vi "TestMotorCommands.vi"() -> ()   [LabVIEW 2017]
uses:
  LV_Source/Subsystems/Motion/DataTypes/Motion Settings--cluster.ctl
  Ichor_Common/Lib/Serial/Comm Channels--cluster.ctl
  Ichor_Common/Lib/Serial/SerialPort Config--cluster.ctl
  Ichor_Common/Lib/SmartMotor/TD SerialBusMotorSpecifier_enum.ctl
  Ichor_Common/Lib/SmartMotor/TD MotorCommands - single motor--enum.ctl
  LV_Source/Subsystems/Motion/Motion.lvclass
panel:
  out "str out 4":string[](array[string])
  out "cmdstr out 4":string[](array[string])
  in  "Rsp?":bool
  out "AdHoc Rsp":string
  in  "AdHoc Cmd":string
  in  "SendAdHoc":bool
  in  "ID":bool
  out "Motor ID":string
  out "str out 3":string[](array[string])
  out "cmdstr out 3":string[](array[string])
  out "str out 2":string[](array[string])
  out "cmdstr out 2":string[](array[string])
  in  "Move":bool
  in  "OK":bool
  in  "MotorSpecifier(None)":T1=enum."M2"
  out "error out":errorcluster
  in  "error in (no error)":errorcluster
  in  "Motion Settings":T2={"Simulate"=FALSE, "SerialPort"=enum."COM3", "SerPort Config"={"termChar"=10, "timeout"=10000, "baud"=9600, "data bits"=8, "parity"=enum."None", "stop bits"=10, "flow control (0:none)"=0}, "MotorStartupCmds"=["€SADDR1", "ECHO", "SLEEP", "€SADDR2", "‚ECHO", "€WAKE"], "EnableTermChar"=FALSE, "MotorSyncTimeout_s"=0.0} {"SerPort Config"."flow control (0:none)" items=["None", "XON/XOFF", "RTS/CTS", "XON/XOFF & RTS/CTS", "DTR/DSR", "XON/XOFF & DTR/DSR"]; "SerPort Config"."stop bits" items=["1.0"=10, "1.5"=15, "2.0"=20]; "SerPort Config"."data bits" min=5 max=8 step=1; "SerPort Config"."termChar" format="%.0x"}
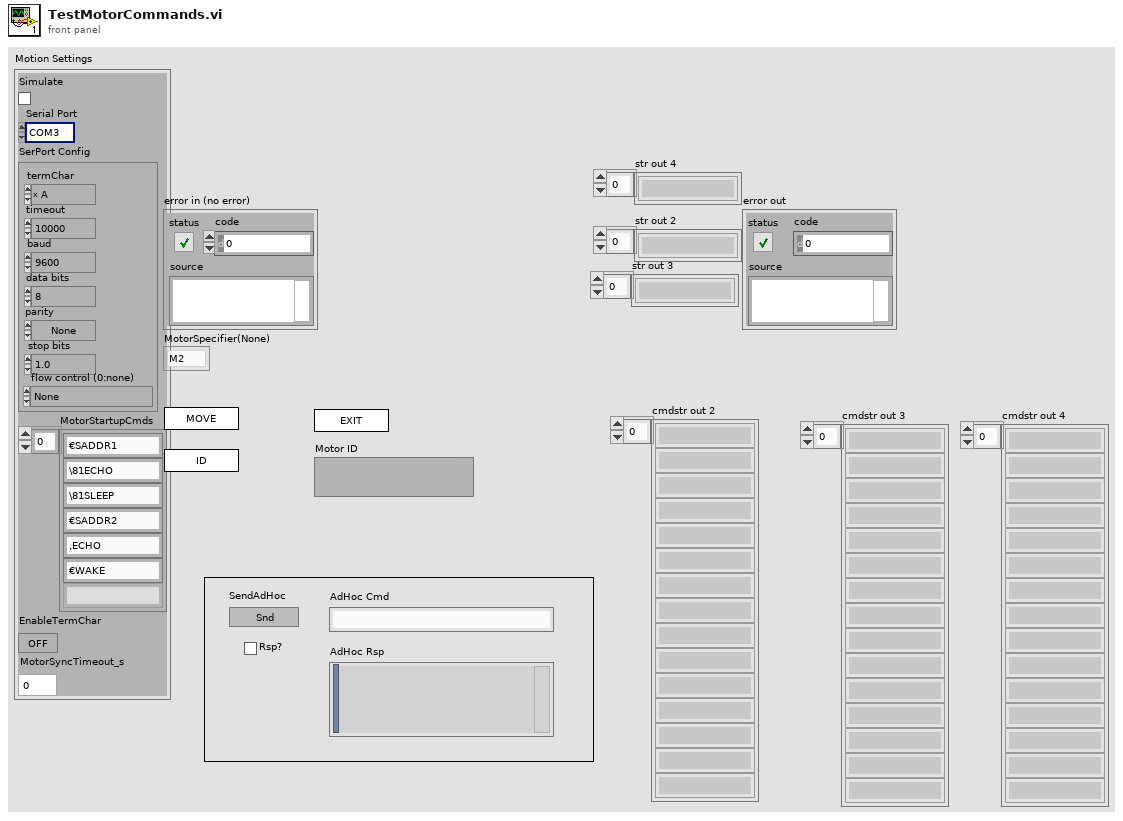
[diagram p1: front panel]
types:
  T1 = typedef "TD SerialBusMotorSpecifier_enum.ctl" = enum16{"None", "Global", "M1", "M2", "M3"}
  T2 = typedef "Motion.lvclass/Motion Settings--cluster.ctl" = cluster{"Simulate":bool, "SerialPort":T3, "SerPort Config":T4, "MotorStartupCmds":string[], "EnableTermChar":bool, "MotorSyncTimeout_s":dbl}
  T3 = typedef "Comm Channels--cluster.ctl" = enum16{"COM1", "COM2", "COM3", "COM4", "COM5", "COM6", "COM7", "COM8", "COM9", "COM10", "COM11", "COM12", "nothing", "LPT1", "LPT2", "LPT3", "LPT4"}
  T4 = typedef "SerialPort Config--cluster.ctl" = cluster{"termChar":u8, "timeout":u32, "baud":u32, "data bits":u16, "parity":enum16{"None", "Odd", "Even", "Mark", "Space"}, "stop bits":u16, "flow control (0:none)":u16}
  T5 = enum32{"invalid app kind", "Development System", "Run Time System", "Student Edition", "Embedded LabVIEW", "Evaluation", "Custom"}
  T6 = enum32{"Invalid", "Standard", "Closed", "Hidden", "Minimized", "Maximized"}
  T7 = typedef "TD MotorCommands - single motor--enum.ctl" = enum16{"Unlisted", "AbortMotion", "StopMotion", "DisableMotor", "ClearErrors", "ZeroEncoder", "SetMode", "GO", "SetEncoder", "En/Ds LmtSwitchs"}
  T8 = cluster{"String Input":string, "ExpectResponse":bool}
  T9 = cluster{"Core":cluster{"Current VI Reference":refnum<vi>, "Close Panel on Exit?":bool}, "VISA":refnum<visa-resource-name>}
  T10 = cluster{"Current VI Reference":refnum<vi>, "Close Panel on Exit?":bool}
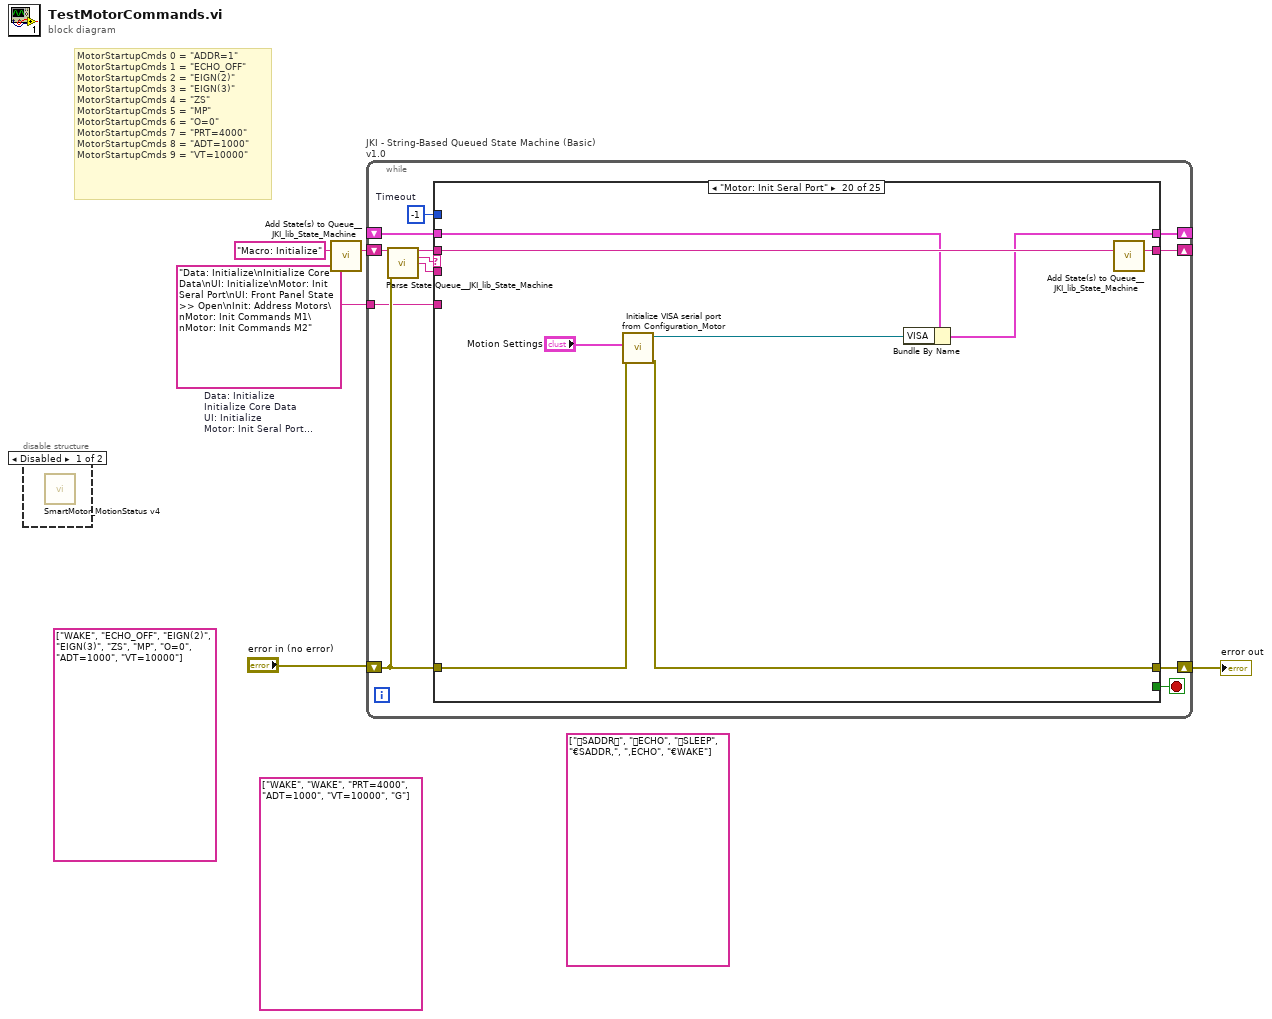
[diagram p0: block diagram]
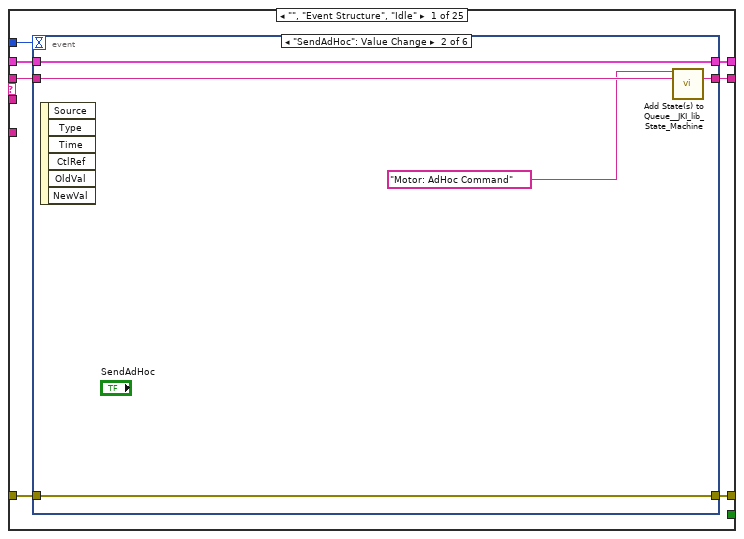
[diagram p3: hidden frame]
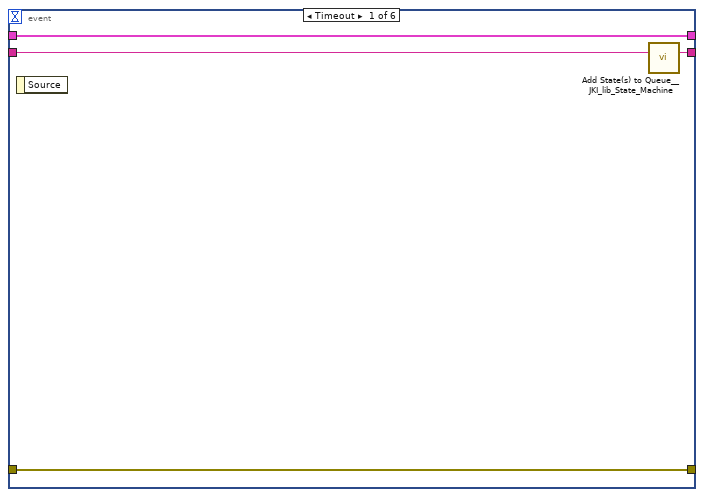
[diagram p4: hidden frame]
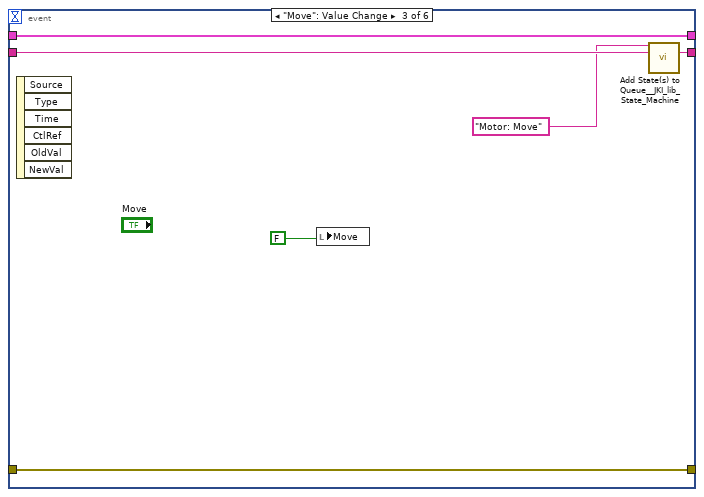
[diagram p5: hidden frame]
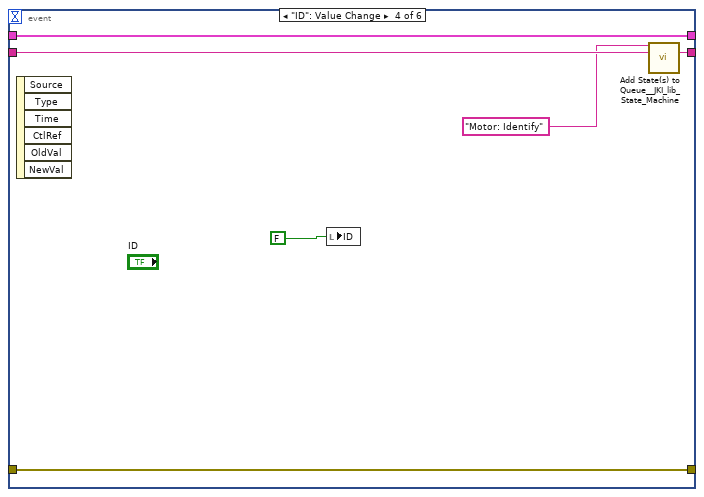
[diagram p6: hidden frame]
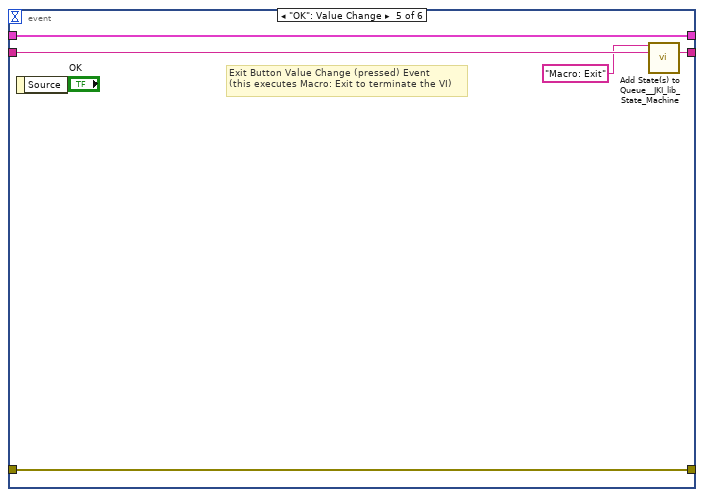
[diagram p7: hidden frame]
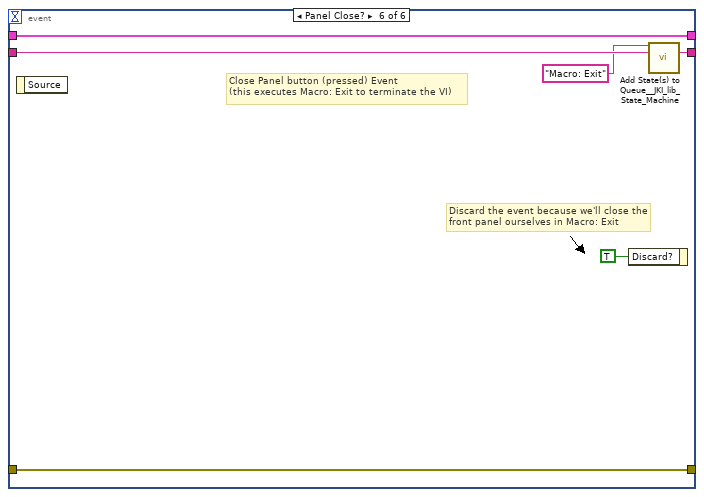
[diagram p8: hidden frame]
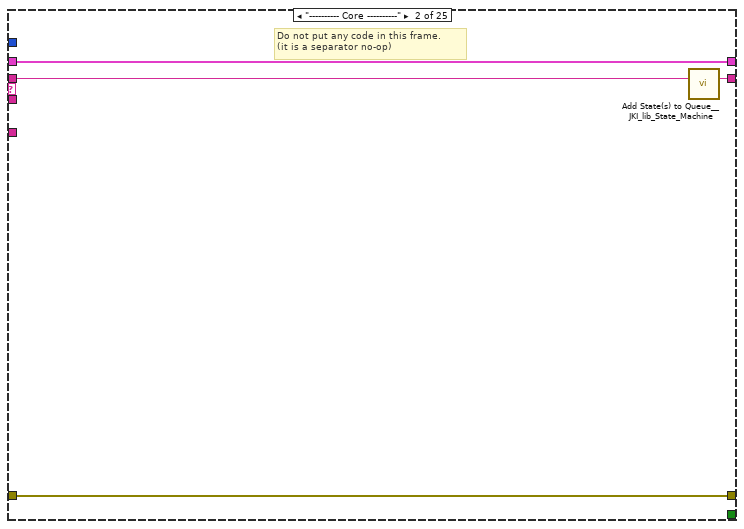
[diagram p9: hidden frame]
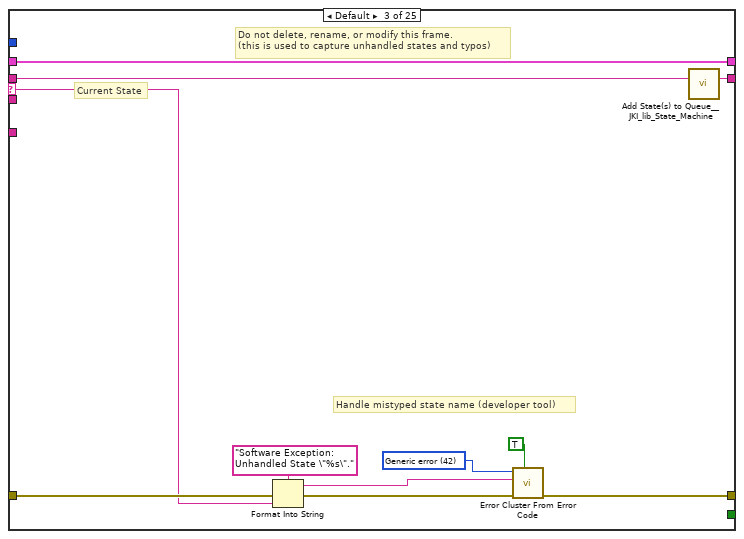
[diagram p10: hidden frame]
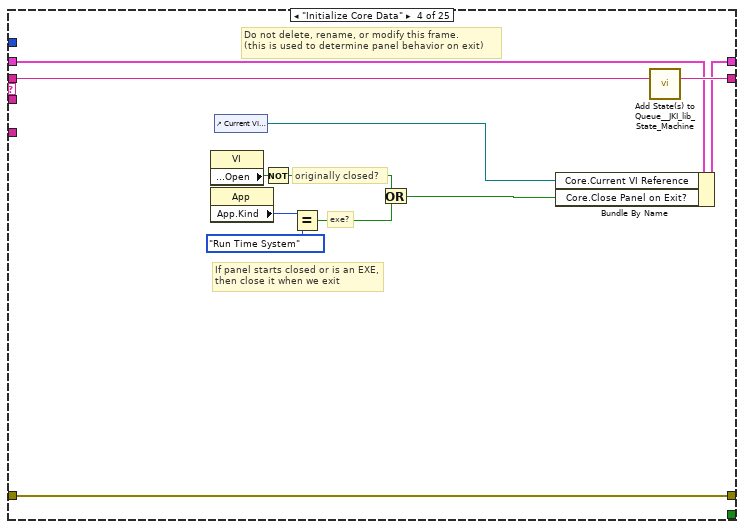
[diagram p11: hidden frame]
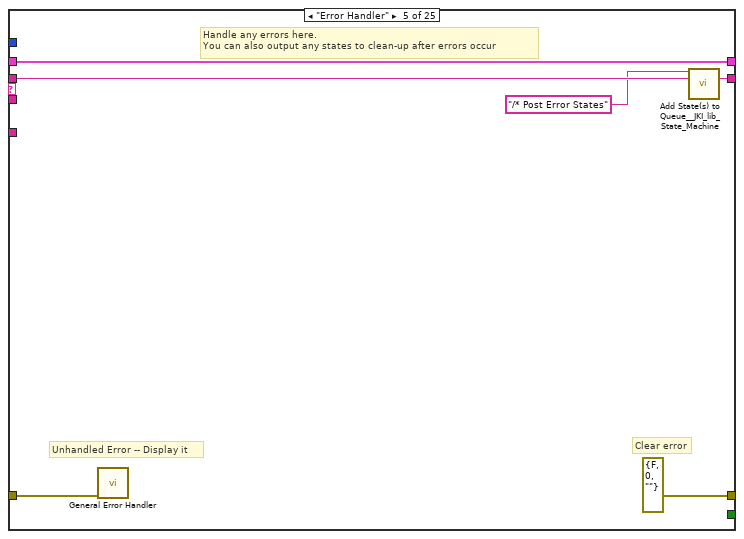
[diagram p12: hidden frame]
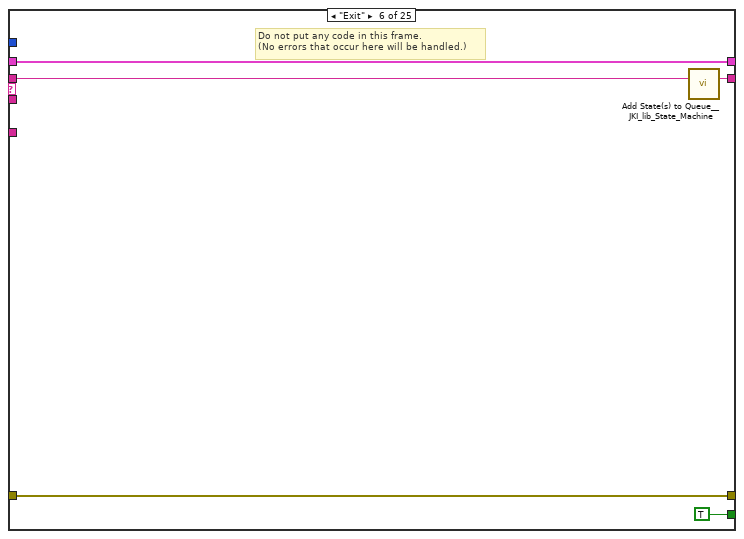
[diagram p13: hidden frame]
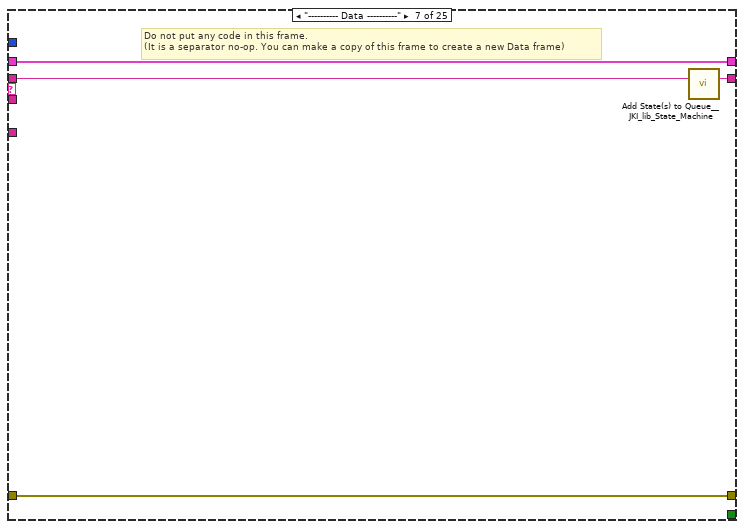
[diagram p14: hidden frame]
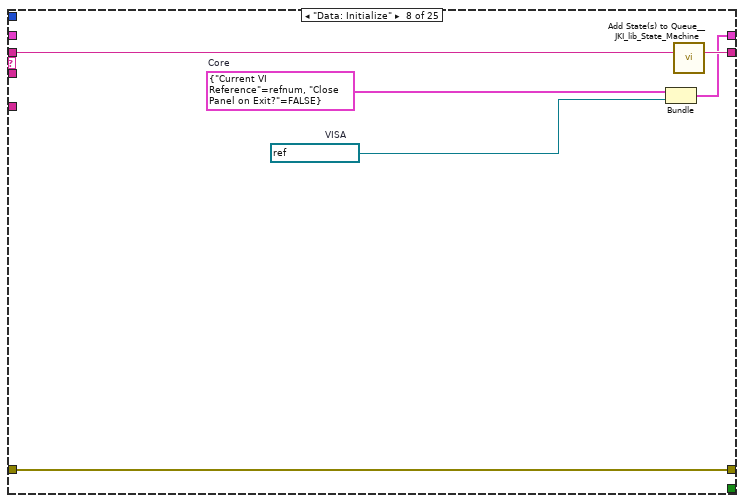
[diagram p15: hidden frame]
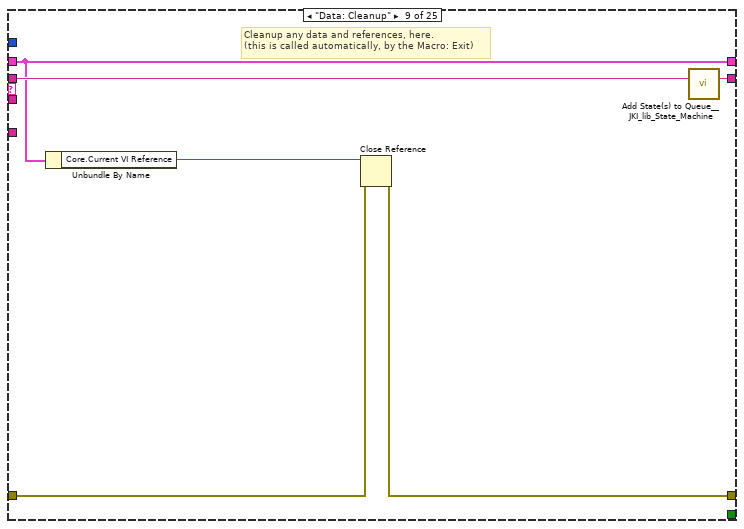
[diagram p16: hidden frame]
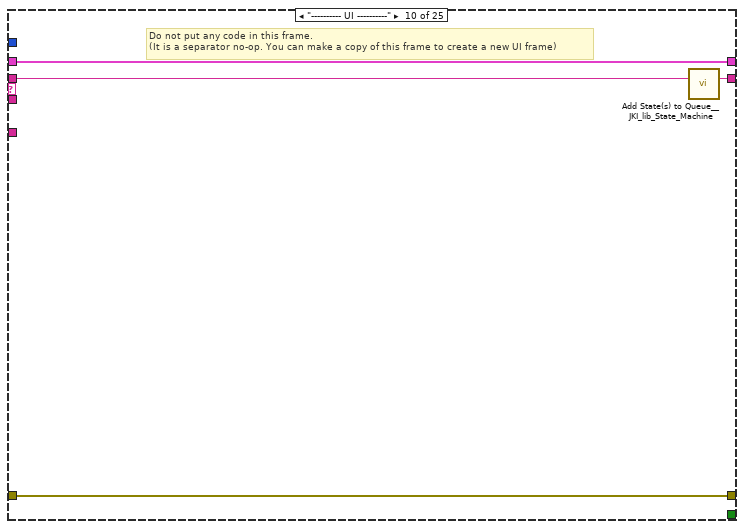
[diagram p17: hidden frame]
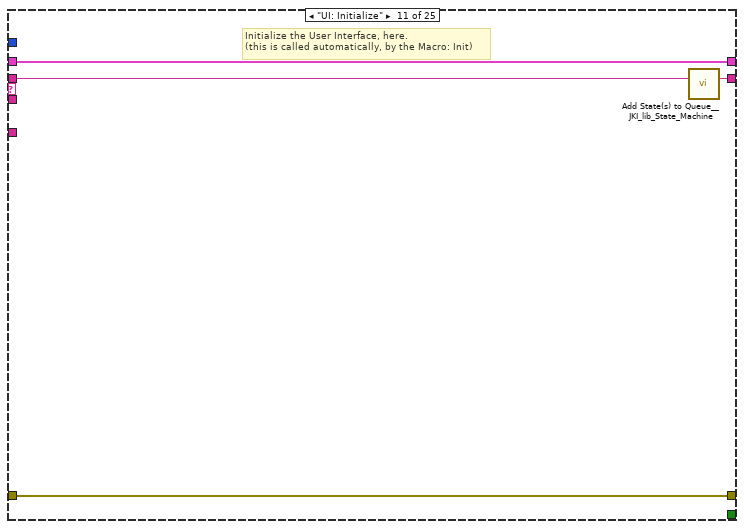
[diagram p18: hidden frame]
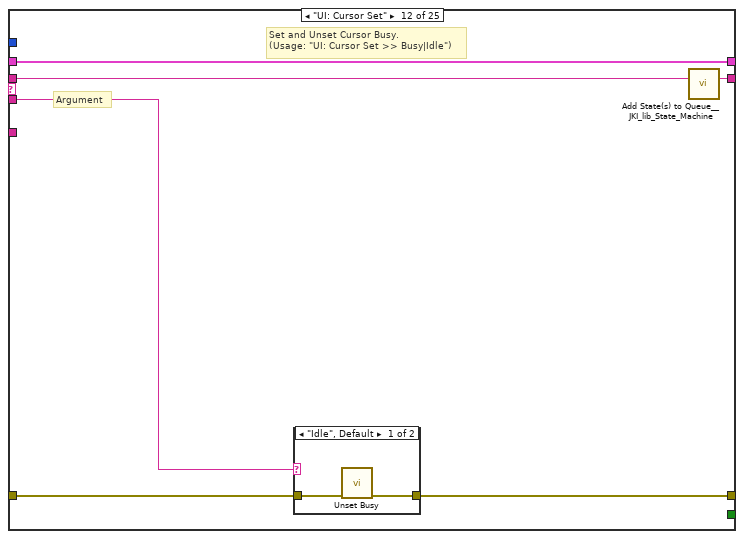
[diagram p19: hidden frame]
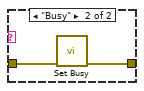
[diagram p20: hidden frame]
diagram:
  (unwired) string[] ["SADDR", "ECHO", "SLEEP", "€SADDR‚", "‚ECHO", "€WAKE"]
  (unwired) string[] ["WAKE", "WAKE", "PRT=4000", "ADT=1000", "VT=10000", "G"]
  (unwired) string[] ["WAKE", "ECHO_OFF", "EIGN(2)", "EIGN(3)", "ZS", "MP", "O=0", "ADT=1000", "VT=10000"]
  w1 = "Data: Initialize\nInitialize Core Data\nUI: Initialize\nMotor: Init Seral Port\nUI: Front Panel State >> Open\nInit: Address Motors\nMotor: Init Commands M1\nMotor: Init Commands M2"  # Data: Initialize Initialize Core Data UI: Initialize Motor: Init Seral Port UI: Front Panel State >> Open Init: Address Motors Motor: Init Commands M1 Motor: Init Commands M2
  # "MotorStartupCmds 0 = \"ADDR=1\"\nMotorStartupCmds 1 = \"ECHO_OFF\"\nMotorStartupCmds 2 = \"EIGN(2)\"\nMotorStartupCmds 3 = \"EIGN(3)\"\nMotorStartupCmds 4 = \"ZS\"\nMotorStartupCmds 5 = \"MP\"\nMotorStartupCmds 6 = \"O=0\"\nMotorStartupCmds 7 = \"PRT=4000\"\nMotorStartupCmds 8 = \"ADT=1000\"\nMotorStartupCmds 9 = \"VT=10000\""
  n1 = disable-structure shown="Disabled" {
    frame Disabled {
      n2 = call "SmartMotor_MotionStatus v4.vi"() -> ()  [unwired: 10 in, 6 out]
    }
    frame Enabled {
    }
  }
  n3 = call <vilib>:"Add State(s) to Queue__JKI_lib_State_Machine.vi"("State(s) in (\"\")"="Macro: Initialize") -> ("States Out"=w5:string)  [unwired: 14 in]
  n4 = while "JKI - String-Based Queued State Machine (Basic) v1.0" {
    shift-right: [w10] -> _
    shift-left: _ -> [w9]
    shift-right: [w13] -> w2
    shift-left: "error in (no error)" -> [w7]
    shift-right: [w12] -> _
    shift-left: w5 -> [w14]
    tunnel: w1 -> [w6]
    stop <- w11 stop-if-true
    w8 = -1  # Timeout
    n5 = call <vilib>:"Parse State Queue__JKI_lib_State_Machine.vi"("State Queue"=w14, "Error In (no error)"=w7) -> ("Remaining States"=w16:string, "Current State"=w17:string, "Arguments"=w15:string)  [unwired: 11 in]
    n6 = case shown="\"Motor: Init Seral Port\"" w17 {
      selector: w17 -> [_ _ w61 _ _ _ _ _ _ _ _ _ _ _ _ _ _ _ _ _ _ _ _ _ _]
      tunnel: w16 -> [w24 w60 w65 w83 w89 w94 w98 w104 w110 w114 w118 w124 w135 w161 w166 w176 w180 w194 w200 w208 w220 w246 w255 w276 w297]
      tunnel: w15 -> [_ _ _ _ _ _ _ _ _ _ _ w119 w129 _ _ _ _ _ _ _ _ _ _ _ _]
      tunnel: w9 -> [w22 w57 w63 w74 w86 w92 w95 _ w105 w111 w116 w122 w131 w158 w163 w173 w177 w192 w196 w205 w213 w241 w250 w271 w292]
      tunnel: [w21 w58 w67 w80 errorcluster {"status"=FALSE, "code"=0, "source"=""} ("error out") w91 w96 w101 w106 w112 w115 w120 w132 w159 w164 w174 w178 w187 w197 w201 w215 w243 w248 w269 w290] -> w13
      tunnel: w7 -> [w20 w58 w66 w80 w85 w91 w96 w101 w107 w112 w115 w121 w133 w159 w164 w174 w178 w188 w198 w202 w214 w242 w247 w268 w289]
      tunnel: [w23 w59 w64 w82 w88 w93 w97 w103 w109 w113 w117 w123 w134 w160 w165 w175 w179 w193 w199 w207 w219 w245 w254 w275 w296] -> w12
      tunnel: [_ _ _ _ _ TRUE _ _ _ _ _ _ _ _ _ _ _ _ _ _ _ _ _ _ _] -> w11
      tunnel: [w19 w57 w63 w81 w86 w92 w95 w102 w105 w111 w116 w122 w131 w158 w163 w173 w177 w192 w196 w204 w212 w240 w250 w271 w292] -> w10
      tunnel: w8 -> [w18 _ _ _ _ _ _ _ _ _ _ _ _ _ _ _ _ _ _ _ _ _ _ _ _]
      tunnel: w6 -> [_ _ _ _ _ _ _ _ _ _ _ _ _ _ w162 _ _ _ _ _ _ _ _ _ _]
      frame "", "Event Structure", "Idle" {
        n7 = event shown="[1] \"SendAdHoc\": Value Change" {
          selector: _ -> [_ _ _ _ _ _]
          dyn-events: _ -> [_ _ _ _ _ _]
          timeout: w18 -> [_ _ _ _ _ _]
          tunnel: w24 -> [w28 w33 w39 w45 w50 w56]
          tunnel: [w27 w32 w38 w44 w49 w55] -> w23
          tunnel: w22 -> [w25 w30 w36 w42 w47 w53]
          tunnel: [w26 w31 w37 w43 w48 w54] -> w21
          tunnel: w20 -> [w26 w31 w37 w43 w48 w54]
          tunnel: [w25 w30 w36 w42 w47 w53] -> w19
          event Timeout {
            n8 = event-data() -> ()  [unwired: 1 in, 1 out]
            n9 = call <vilib>:"Add State(s) to Queue__JKI_lib_State_Machine.vi"("State(s) in (\"\")"=w28) -> ("States Out"=w27:string)  [unwired: 14 in]
          }
          event "SendAdHoc": Value Change {
            n10 = event-data() -> ()  [unwired: 1 in, 6 out]
            n11 = call <vilib>:"Add State(s) to Queue__JKI_lib_State_Machine.vi"("State(s) in Front (\"\")"="Motor: AdHoc Command", "State(s) in (\"\")"=w33) -> ("States Out"=w32:string)  [unwired: 13 in]
          }
          event "Move": Value Change {
            n12 = event-data() -> ()  [unwired: 1 in, 6 out]
            n13 = local write "Move"(FALSE ("Move")) -> ()
            n14 = call <vilib>:"Add State(s) to Queue__JKI_lib_State_Machine.vi"("State(s) in Front (\"\")"="Motor: Move" ("State(s) in Front (\"\")"), "State(s) in (\"\")"=w39) -> ("States Out"=w38:string)  [unwired: 13 in]
          }
          event "ID": Value Change {
            n15 = event-data() -> ()  [unwired: 1 in, 6 out]
            n16 = local write "ID"(FALSE ("Move")) -> ()
            n17 = call <vilib>:"Add State(s) to Queue__JKI_lib_State_Machine.vi"("State(s) in Front (\"\")"="Motor: Identify" ("State(s) in Front (\"\")"), "State(s) in (\"\")"=w45) -> ("States Out"=w44:string)  [unwired: 13 in]
          }
          event "OK": Value Change {
            # "Exit Button Value Change (pressed) Event\n(this executes Macro: Exit to terminate the VI)"
            n18 = event-data() -> ()  [unwired: 1 in, 1 out]
            n19 = call <vilib>:"Add State(s) to Queue__JKI_lib_State_Machine.vi"("State(s) in Front (\"\")"="Macro: Exit", "State(s) in (\"\")"=w50) -> ("States Out"=w49:string)  [unwired: 13 in]
          }
          event Panel Close? {
            # "Discard the event because we'll close the front panel ourselves in Macro: Exit"
            # "Close Panel button (pressed) Event\n(this executes Macro: Exit to terminate the VI)"
            n20 = event-data() -> ()  [unwired: 1 in, 1 out]
            n21 = event-data("Discard?"=TRUE) -> ()  [unwired: 1 in, 1 out]
            n22 = call <vilib>:"Add State(s) to Queue__JKI_lib_State_Machine.vi"("State(s) in Front (\"\")"="Macro: Exit", "State(s) in (\"\")"=w56) -> ("States Out"=w55:string)  [unwired: 13 in]
          }
        }
      }
      frame "---------- Core ----------" {
        # "Do not put any code in this frame.\n(it is a separator no-op)"
        n23 = call <vilib>:"Add State(s) to Queue__JKI_lib_State_Machine.vi"("State(s) in (\"\")"=w60) -> ("States Out"=w59:string)  [unwired: 14 in]
      }
      frame Default {
        w70 = 42 items=["No error", "Argument error", "Memory is full", "Out of zone", "End of file", "File already open", "Generic file I/O error", "File not found", "File permission error", "Disk is full", "Duplicate path", "Too many files open", "System feature not enabled", "Resource file not found", "Cannot add resource", "Resource not found", "Image not found", "Image memory error", "Pen does not exist", "Config type invalid", "Config token not found", "Config parse error", "Config memory error", "Bad external code format", "Bad external code offset", "External code not present", "Null window", "Destroy window error", "Null menu", "Print aborted", "Bad print record", "Print driver error", "Windows error during printing", "Memory error during printing", "Print dialog error", "Generic print error", "Invalid device refnum", "Device not found", "Device parameter error", "Device unit error", "Cannot open device", "Device call aborted", "Generic error", "Cancelled by user", "Object ID too low", "Object ID too high", "Object not in heap", "Unknown heap", "Unknown object (invalid DefProc)", "Unknown object (DefProc not in table)", "Message out of range", "Invalid (null) method", "Unknown message", "Manager call not supported", "Bad address", "Network operation in progress", "Network operation timed out", "Connection is busy", "Network attribute not supported", "Network error", "Address in use", "System out of memory", "Connection aborted", "Connection refused", "Not connected", "Already connected", "Connection closed", "Initialization error (interapplication manager)", "Bad occurrence", "Wait on unbound occurrence handler", "Occurrence queue overflow", "Datalog type conflict", "Unused", "Unrecognized type (interapplication manager)", "Memory corrupt", "Failed to make temporary DLL", "Old CIN version", "Drag socket not found", "Failed to load drop-object", "Failed to register OLE object", "Failed to release OLE object", "Format specifier type mismatch", "Unknown format specifier", "Too few format specifiers", "Too many format specifiers", "Scan failed", "Newer CIN version", "Error converting to variant", "Runtime menu error", "Password tampered", "Variant attribute not found", "Incompatible variant data type", "Event data is not available", "Event Store is not present", "Occurrence is not found", "Event Queue is not created", "Event info is not available", "Refnum passed is NULL", "Error retrieving Class GUID", "Error retrieving CoClass GUID", "Error retrieving TypeLib GUID.", "Bad built application magic bytes.", "Specific driver is different from the specific driver associated with the Logical Name.", "There is no session opened to the class driver.", "Max Error", "MAX - Error with config objects", "MAX - Error loading configuration", "MAX - Group not supported"]
        # "Current State"
        # "Do not delete, rename, or modify this frame.\n(this is used to capture unhandled states and typos)"
        # "Handle mistyped state name (developer tool)"
        n24 = Format Into String(format string="Software Exception: Unhandled State \"%s\"." ("message"), error in=w66, w61) -> (resulting string=w69:string, error out=w68:errorcluster)  [unwired: 1 in]
        n25 = call <vilib>:"Error Cluster From Error Code.vi"("show call chain? (False)"=TRUE, "error in (no error)"=w68, "error message (\"\")"=w69, "error code (0)"=w70) -> ("error out"=w67:errorcluster)  [unwired: 5 in]
        n26 = call <vilib>:"Add State(s) to Queue__JKI_lib_State_Machine.vi"("State(s) in (\"\")"=w65) -> ("States Out"=w64:string)  [unwired: 14 in]
      }
      frame "Initialize Core Data" {
        # "Do not delete, rename, or modify this frame.\n(this is used to determine panel behavior on exit)"
        # "originally closed?"
        # "exe?"
        # "If panel starts closed or is an EXE, then close it when we exit"
        n27 = property class="VI"() -> ("Front Panel.Open"=w79:bool)  [unwired: 2 in, 2 out]
        n28 = property class="App"() -> ("App.Kind"=w78:T5)  [unwired: 2 in, 2 out]
        n29 = control-ref of="Current VI Reference"() -> (w72:refnum<vi>)
        n30 = Not(x=w79) -> (.not. x?=w76:bool)
        n31 = Equal?(x=w78, y=T5."Run Time System" ("Application:Kind")) -> (x = y?=w75:bool)
        n32 = Or(x=w76, y=w75) -> (x .or. y?=w73:bool)
        n33 = Bundle By Name(cluster=w74, "Core.Current VI Reference"=w72, "Core.Close Panel on Exit?"=w73) -> (w81:T9)
        n34 = call <vilib>:"Add State(s) to Queue__JKI_lib_State_Machine.vi"("State(s) in (\"\")"=w83) -> ("States Out"=w82:string)  [unwired: 14 in]
      }
      frame "Error Handler" {
        # "Unhandled Error -- Display it"
        # "Handle any errors here.\nYou can also output any states to clean-up after errors occur"
        # "Clear error"
        n35 = call <vilib>:"General Error Handler.vi"("error in (no error)"=w85) -> ()  [unwired: 10 in, 5 out]
        n36 = call <vilib>:"Add State(s) to Queue__JKI_lib_State_Machine.vi"("State(s) in Front (\"\")"="/* Post Error States", "State(s) in (\"\")"=w89) -> ("States Out"=w88:string)  [unwired: 13 in]
      }
      frame "Exit" {
        # "Do not put any code in this frame.\n(No errors that occur here will be handled.)"
        n37 = call <vilib>:"Add State(s) to Queue__JKI_lib_State_Machine.vi"("State(s) in (\"\")"=w94) -> ("States Out"=w93:string)  [unwired: 14 in]
      }
      frame "---------- Data ----------" {
        # "Do not put any code in this frame.\n(It is a separator no-op. You can make a copy of this frame to create a new Data frame)"
        n38 = call <vilib>:"Add State(s) to Queue__JKI_lib_State_Machine.vi"("State(s) in (\"\")"=w98) -> ("States Out"=w97:string)  [unwired: 14 in]
      }
      frame "Data: Initialize" {
        w99 = refnum<visa-resource-name> "COM3"  # VISA
        w100 = T10 {"Current VI Reference"=refnum, "Close Panel on Exit?"=FALSE}  # Core
        n39 = Bundle("Core"=w100, "VISA"=w99) -> (w102:T9)  [unwired: 1 in]
        n40 = call <vilib>:"Add State(s) to Queue__JKI_lib_State_Machine.vi"("State(s) in (\"\")"=w104) -> ("States Out"=w103:string)  [unwired: 14 in]
      }
      frame "Data: Cleanup" {
        # "Cleanup any data and references, here.\n(this is called automatically, by the Macro: Exit)"
        n41 = Unbundle By Name(w105) -> ("Core.Current VI Reference"=w108:refnum<vi>)
        n42 = Close Reference(reference=w108, error in (no error)=w107) -> (error out=w106:errorcluster)
        n43 = call <vilib>:"Add State(s) to Queue__JKI_lib_State_Machine.vi"("State(s) in (\"\")"=w110) -> ("States Out"=w109:string)  [unwired: 14 in]
      }
      frame "---------- UI ----------" {
        # "Do not put any code in this frame.\n(It is a separator no-op. You can make a copy of this frame to create a new UI frame)"
        n44 = call <vilib>:"Add State(s) to Queue__JKI_lib_State_Machine.vi"("State(s) in (\"\")"=w114) -> ("States Out"=w113:string)  [unwired: 14 in]
      }
      frame "UI: Initialize" {
        # "Initialize the User Interface, here.\n(this is called automatically, by the Macro: Init)"
        n45 = call <vilib>:"Add State(s) to Queue__JKI_lib_State_Machine.vi"("State(s) in (\"\")"=w118) -> ("States Out"=w117:string)  [unwired: 14 in]
      }
      frame "UI: Cursor Set" {
        # "Argument"
        # "Set and Unset Cursor Busy.\n(Usage: \"UI: Cursor Set >> Busy|Idle\")"
        n46 = case shown="\"Idle\", Default" w119 {
          tunnel: w121 -> [w126 w128]
          tunnel: [w125 w127] -> w120
          frame "Idle", Default {
            n47 = call <vilib>:"Unset Busy.vi"("error in (no error)"=w126) -> ("error out"=w125:errorcluster)  [unwired: 10 in]
          }
          frame "Busy" {
            n48 = call <vilib>:"Set Busy.vi"("error in (no error)"=w128) -> ("error out"=w127:errorcluster)  [unwired: 9 in, 1 out]
          }
        }
        n49 = call <vilib>:"Add State(s) to Queue__JKI_lib_State_Machine.vi"("State(s) in (\"\")"=w124) -> ("States Out"=w123:string)  [unwired: 14 in]
      }
      frame "UI: Front Panel State" {
        # "Argument"
        # "Set Front Panel Open or Closed\n(Usage: \"UI: Front Panel State >> Open|Close\")"
        n50 = Unbundle By Name(w131) -> ("Core.Current VI Reference"=w130:refnum<vi>)
        n51 = case shown="\"Open\", Default" w129 {
          tunnel: w133 -> [w139 w152]
          tunnel: [w141 w153] -> w132
          tunnel: w130 -> [w140 w150]
          frame "Open", Default {
            n52 = property class="VI"(reference=w140, error in=w139) -> (reference out=w137:refnum<vi>, error out=w138:errorcluster, "Front Panel.Open"=w136:bool)
            n53 = case shown="False" w136 {
              tunnel: [w144 w147] -> w141
              tunnel: w138 -> [w143 w147]
              tunnel: w137 -> [w142 _]
              frame False {
                n54 = invoke class="VI" method="FP.Open"(reference=w142, error in=w143, "Activate"=TRUE, "State"=T6."Standard") -> (error out=w144:errorcluster)  [unwired: 1 in, 4 out]
              }
              frame True {
              }
            }
          }
          frame "Close" {
            n55 = property class="VI"(reference=w150, error in=w152) -> (reference out=w149:refnum<vi>, error out=w151:errorcluster, "Front Panel.Open"=w148:bool)
            n56 = case shown="True" w148 {
              tunnel: [w154 w157] -> w153
              tunnel: w151 -> [w154 w156]
              tunnel: w149 -> [_ w155]
              frame False {
              }
              frame True {
                n57 = invoke class="VI" method="FP.Close"(reference=w155, error in=w156) -> (error out=w157:errorcluster)  [unwired: 1 in, 2 out]
              }
            }
          }
        }
        n58 = call <vilib>:"Add State(s) to Queue__JKI_lib_State_Machine.vi"("State(s) in (\"\")"=w135) -> ("States Out"=w134:string)  [unwired: 14 in]
      }
      frame "---------- Macro ----------" {
        # "Do not put any code in this frame.\n(It is a separator no-op. You can make a copy of this frame to create a new Macro frame)"
        n59 = call <vilib>:"Add State(s) to Queue__JKI_lib_State_Machine.vi"("State(s) in (\"\")"=w161) -> ("States Out"=w160:string)  [unwired: 14 in]
      }
      frame "Macro: Initialize" {
        # "Initialization Macro\n(This is called once, when the VI starts)"
        n60 = call <vilib>:"Add State(s) to Queue__JKI_lib_State_Machine.vi"("State(s) in Front (\"\")"=w162, "State(s) in (\"\")"=w166) -> ("States Out"=w165:string)  [unwired: 13 in]
      }
      frame "Macro: Exit" {
        # "Exit Macro\n(This is called once, when the VI exits)"
        n61 = Unbundle By Name(w173) -> ("Core.Close Panel on Exit?"=w172:bool)
        n62 = Select(t="UI: Front Panel State >> Close", s=w172, f="") -> (s? t:f=w169:string)
        n63 = call <vilib>:"Add State(s) to Queue__JKI_lib_State_Machine.vi"("State(s) in (\"\")"=w169, "State(s) at Back (\"\")"="Motor: Close\nData: Cleanup\nExit") -> ("States Out"=w167:string)  [unwired: 13 in]
        n64 = call <vilib>:"Add State(s) to Queue__JKI_lib_State_Machine.vi"("State(s) in Front (\"\")"=w167, "State(s) in (\"\")"=w176) -> ("States Out"=w175:string)  [unwired: 13 in]
      }
      frame "---------- Motor ----------" {
        # "Template Separator\n(You can make a copy of, or modify, this frame)"
        n65 = call <vilib>:"Add State(s) to Queue__JKI_lib_State_Machine.vi"("State(s) in (\"\")"=w180) -> ("States Out"=w179:string)  [unwired: 14 in]
      }
      frame "Motor: AdHoc Command" {
        # "Template Separator\n(You can make a copy of, or modify, this frame)"
        n66 = Bundle By Name(cluster=T8 {"String Input"="", "ExpectResponse"=FALSE} ("Adhoc Input"), "String Input"="AdHoc Cmd", "ExpectResponse"="Rsp?") -> (w182:T8)
        n67 = local read "MotorSpecifier(None)"() -> (w190:T1)
        n68 = Unbundle By Name(w192) -> ("VISA"=w191:refnum<visa-resource-name>)
        n69 = call "SmartMotor_SendCommand - single motor.vi"("VISA In"=w191, "MotorCmd"=TD_MotorCommands_-_single_motor--enum."Unlisted", "Adhoc Input"=w182, "MotorSpecifier(M1)"=w190, "Read wait (ms)"=u32 20, "error in"=w188) -> ("Response Str"=→"AdHoc Rsp":string, "error out"=w187:errorcluster)  [unwired: 6 in, 2 out]
        n70 = call <vilib>:"Add State(s) to Queue__JKI_lib_State_Machine.vi"("State(s) in (\"\")"=w194) -> ("States Out"=w193:string)  [unwired: 14 in]
      }
      frame "Motor: Close" {
        n71 = Unbundle By Name(w196) -> ("VISA"=w195:refnum<visa-resource-name>)
        n72 = VISA Close(VISA resource name=w195, error in (no error)=w198) -> (error out=w197:errorcluster)
        n73 = call <vilib>:"Add State(s) to Queue__JKI_lib_State_Machine.vi"("State(s) in (\"\")"=w200) -> ("States Out"=w199:string)  [unwired: 14 in]
      }
      frame "Motor: Init Seral Port" {
        n74 = call "Initialize VISA serial port from Configuration_Motor.vi"("error in (no error)"=w202, "MotionConfig"="Motion Settings") -> ("error out"=w201:errorcluster, "VISA Out"=w203:refnum<visa-resource-name>)  [unwired: 7 in, 1 out]
        n75 = Bundle By Name(cluster=w205, "VISA"=w203) -> (w204:T9)
        n76 = call <vilib>:"Add State(s) to Queue__JKI_lib_State_Machine.vi"("State(s) in (\"\")"=w208) -> ("States Out"=w207:string)  [unwired: 14 in]
      }
      frame "Motor: Move" {
        # "Your code here.\n(You can make a copy of, or modify, this frame)"
        n77 = Unbundle By Name(w213) -> ("VISA"=w216:refnum<visa-resource-name>)
        n78 = for {
          shift-right: [w230] -> w211
          shift-left: w216 -> [w231]
          tunnel: string[] ["O=0", "PRT=4000", "G"] -> [w229] mode=indexing
          shift-right: [w222] -> w215
          shift-left: w214 -> [w228]
          tunnel: "MotorSpecifier(None)" -> [w226]
          tunnel: [w225] -> w210 mode=indexing
          tunnel: [w224] -> w209 mode=indexing
          n79 = call "SmartMotor_serial cmd-response.vi"("VISA In"=w231, "mode"=enum16{"wr & rd", "write", "read"}."write", "cmd"=w229, "error in"=w228, "Sem Timeout (5000)"=5000, "MotorSpecifier(None)"=w226) -> ("VISA out"=w230:refnum<visa-resource-name>, "str out"=w225:string, "cmd str out"=w224:string, "error out"=w223:errorcluster)  [unwired: 5 in, 1 out]
          n80 = local write "error out"(w223) -> ()
          n81 = call <userlib>:"Wait (ms)__ogtk.vi"("error in (no error)"=w223, "milliseconds to wait"=u32 100) -> ("error out"=w222:errorcluster)  [unwired: 8 in, 1 out]
        }
        n82 = local write "cmdstr out 2"(w209) -> ()
        n83 = Bundle By Name(cluster=w213, "VISA"=w211) -> (w212:T9)
        n84 = local write "str out 2"(w210) -> ()
        n85 = call <vilib>:"Add State(s) to Queue__JKI_lib_State_Machine.vi"("State(s) in (\"\")"=w220) -> ("States Out"=w219:string)  [unwired: 14 in]
      }
      frame "Motor: Identify" {
        n86 = property on="MotorSpecifier(None)" class="Enum (strict)"() -> ("Value"=w234:T1)  [unwired: 2 in, 2 out]
        n87 = Unbundle By Name(w241) -> ("VISA"=w244:refnum<visa-resource-name>)
        n88 = call "SmartMotor_serial cmd-response.vi"("VISA In"=w244, "mode"=enum16{"wr & rd", "write", "read"}."wr & rd", "cmd"="IDENT", "Read wait (20ms)"=u32 200, "error in"=w242, "Sem Timeout (5000)"=5000, "MotorSpecifier(None)"=w234) -> ("VISA out"=w239:refnum<visa-resource-name>, "str out"=→"Motor ID":string, "error out"=w243:errorcluster)  [unwired: 4 in, 2 out]
        n89 = local write "error out"(w243) -> ()
        n90 = Bundle By Name(cluster=w241, "VISA"=w239) -> (w240:T9)
        n91 = call <vilib>:"Add State(s) to Queue__JKI_lib_State_Machine.vi"("State(s) in (\"\")"=w246) -> ("States Out"=w245:string)  [unwired: 14 in]
      }
      frame "Motor: Init Commands M1" {
        n92 = Unbundle By Name(w250) -> ("VISA"=w249:refnum<visa-resource-name>)
        n93 = for {
          shift-right: [w265] -> _
          shift-left: w249 -> [w266]
          tunnel: string[] ["ECHO", "EIGN(2)", "EIGN(3)", "ZS", "MP", "O=0", "ADT=1000", "VT=10000"] -> [w264] mode=indexing
          shift-right: [w258] -> w248
          shift-left: w247 -> [w263]
          tunnel: [w262] -> w252 mode=indexing
          tunnel: [w261] -> w253 mode=indexing
          n94 = call "SmartMotor_serial cmd-response.vi"("VISA In"=w266, "mode"=enum16{"wr & rd", "write", "read"}."write", "cmd"=w264, "error in"=w263, "Sem Timeout (5000)"=5000, "MotorSpecifier(None)"=TD_SerialBusMotorSpecifier_enum."M1" ("MotorSpecifier(None) 2")) -> ("VISA out"=w265:refnum<visa-resource-name>, "str out"=w262:string, "cmd str out"=w261:string, "error out"=w259:errorcluster)  [unwired: 5 in, 1 out]
          n95 = local write "error out"(w259) -> ()
          n96 = call <userlib>:"Wait (ms)__ogtk.vi"("error in (no error)"=w259, "milliseconds to wait"=u32 50) -> ("error out"=w258:errorcluster)  [unwired: 8 in, 1 out]
        }
        "str out 2" <- w252
        "cmdstr out 2" <- w253
        n97 = call <vilib>:"Add State(s) to Queue__JKI_lib_State_Machine.vi"("State(s) in (\"\")"=w255) -> ("States Out"=w254:string)  [unwired: 14 in]
      }
      frame "Init: Address Motors" {
        n98 = Unbundle By Name(w271) -> ("VISA"=w270:refnum<visa-resource-name>)
        n99 = for {
          shift-right: [w286] -> _
          shift-left: w270 -> [w287]
          tunnel: string[] ["€SADDR1", "ECHO", "SLEEP", "€SADDR2", "‚ECHO", "€WAKE"] -> [w285] mode=indexing
          shift-right: [w279] -> w269
          shift-left: w268 -> [w284]
          tunnel: [w283] -> w273 mode=indexing
          tunnel: [w282] -> w274 mode=indexing
          n100 = call "SmartMotor_serial cmd-response.vi"("VISA In"=w287, "mode"=enum16{"wr & rd", "write", "read"}."write", "cmd"=w285, "error in"=w284, "Sem Timeout (5000)"=5000, "MotorSpecifier(None)"=TD_SerialBusMotorSpecifier_enum."None" ("MotorSpecifier(None) 2")) -> ("VISA out"=w286:refnum<visa-resource-name>, "str out"=w283:string, "cmd str out"=w282:string, "error out"=w280:errorcluster)  [unwired: 5 in, 1 out]
          n101 = local write "error out"(w280) -> ()
          n102 = call <userlib>:"Wait (ms)__ogtk.vi"("error in (no error)"=w280, "milliseconds to wait"=u32 50) -> ("error out"=w279:errorcluster)  [unwired: 8 in, 1 out]
        }
        "str out 4" <- w273
        "cmdstr out 4" <- w274
        n103 = call <vilib>:"Add State(s) to Queue__JKI_lib_State_Machine.vi"("State(s) in (\"\")"=w276) -> ("States Out"=w275:string)  [unwired: 14 in]
      }
      frame "Motor: Init Commands M2" {
        n104 = Unbundle By Name(w292) -> ("VISA"=w291:refnum<visa-resource-name>)
        n105 = for {
          shift-right: [w307] -> _
          shift-left: w291 -> [w308]
          tunnel: string[] ["ECHO", "EIGN(2)", "EIGN(3)", "ZS", "MP", "O=0", "ADT=1000", "VT=10000"] -> [w306] mode=indexing
          shift-right: [w300] -> w290
          shift-left: w289 -> [w305]
          tunnel: [w304] -> w294 mode=indexing
          tunnel: [w303] -> w295 mode=indexing
          n106 = call "SmartMotor_serial cmd-response.vi"("VISA In"=w308, "mode"=enum16{"wr & rd", "write", "read"}."write", "cmd"=w306, "error in"=w305, "Sem Timeout (5000)"=5000, "MotorSpecifier(None)"=TD_SerialBusMotorSpecifier_enum."M2") -> ("VISA out"=w307:refnum<visa-resource-name>, "str out"=w304:string, "cmd str out"=w303:string, "error out"=w301:errorcluster)  [unwired: 5 in, 1 out]
          n107 = local write "error out"(w301) -> ()
          n108 = call <userlib>:"Wait (ms)__ogtk.vi"("error in (no error)"=w301, "milliseconds to wait"=u32 100) -> ("error out"=w300:errorcluster)  [unwired: 8 in, 1 out]
        }
        "str out 3" <- w294
        "cmdstr out 3" <- w295
        n109 = call <vilib>:"Add State(s) to Queue__JKI_lib_State_Machine.vi"("State(s) in (\"\")"=w297) -> ("States Out"=w296:string)  [unwired: 14 in]
      }
    }
  }
  "error out" <- w2
